vi "Condition ROI data.vi"(8 "error in (no error)":errorcluster, 9 "ROI numbers":i32[](array[numeric]), 10 "Data for ticked ROI":T1=[{"Plot.Plot Name"="1: Point", "Data"={"X-Axis values"=array[43860 elements], "Y-Axis values (s)"=array[43860 elements]}, "Timeline data"={"X-Axis values"=[], "Y-Axis values (s)"=[]}, "Type"=enum."Mini-scan", "Points per cycle"=1, "ROI number"=0}]) -> (0 "error out":errorcluster, 2 "Sorted Pointers":i32[](array[numeric]), 3 "Data reference":refnum<data-value>)   [LabVIEW 2013]
uses:
  xcontrol/Interface VIs/Interface typedefs/Interface-Data array.ctl
  xcontrol/Interface VIs/Interface typedefs/Interface-Data format definition.ctl
  xcontrol/Typedefs/Xctl-XY data type definition.ctl
  xcontrol/Typedefs/Xctrl-ROI type enum.ctl
  xcontrol/XGrapher.xctl
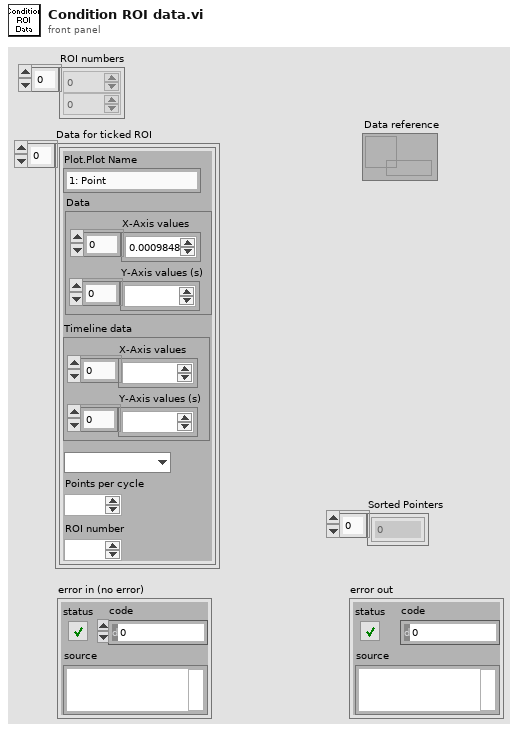
[diagram p1: front panel]
types:
  T1 = typedef "Interface-Data array.ctl" = T2[]
  T2 = typedef "Interface-Data format definition.ctl" = cluster{"Plot.Plot Name":string, "Data":T3, "Timeline data":T3, "Type":T4, "Points per cycle":u16, "ROI number":u16}
  T3 = typedef "XGrapher.xctl/Xctl-XY data type definition.ctl" = cluster{"X-Axis values":sgl[], "Y-Axis values (s)":i32[]}
  T4 = typedef "Xctrl-ROI type enum.ctl" = enum16{"POI", "Mini-scan", "Group"}
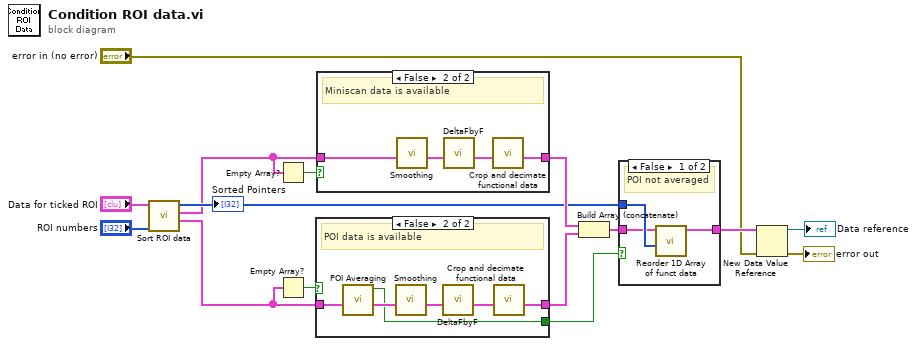
[diagram p0: block diagram]
diagram:
  n1 = call "Sort ROI data.vi"("ROI numbers"="ROI numbers", "Data for ticked ROI"="Data for ticked ROI") -> ("POI raw data"=w4:T1, "Miniscan raw data"=w3:T1, "Sorted Pointers"=w5:i32[])  [unwired: 7 in]
  "Sorted Pointers" <- w5
  n2 = Empty Array?(array=w3) -> (empty?=w11:bool)
  n3 = Empty Array?(array=w4) -> (empty?=w10:bool)
  n4 = case shown="False" w10 {
    tunnel: w4 -> [w16 w20]
    tunnel: [w16 w17] -> w13
    tunnel: [_ w19] -> w15
    frame True {
      # "No POI data available"
    }
    frame False {
      # "POI data is available"
      n5 = call "POI Averaging.vi"("Data in"=w20) -> ("Data out"=w21:T1, "Averaged"=w19:bool)  [unwired: 9 in]
      n6 = call "Smoothing.vi"("Data in"=w21) -> ("Data out"=w22:T1)  [unwired: 10 in]
      n7 = call "DeltaFbyF.vi"("Data in"=w22) -> ("Data out"=w18:T1)  [unwired: 10 in]
      n8 = call "Crop and decimate functional data.vi"("Data in"=w18) -> ("Data out"=w17:T1)  [unwired: 10 in]
    }
  }
  n9 = case shown="False" w11 {
    tunnel: w3 -> [w23 w26]
    tunnel: [w23 w24] -> w12
    frame True {
      # "No miniscan data available"
    }
    frame False {
      # "Miniscan data is available"
      n10 = call "Smoothing.vi"("Data in"=w26) -> ("Data out"=w27:T1)  [unwired: 10 in]
      n11 = call "DeltaFbyF.vi"("Data in"=w27) -> ("Data out"=w25:T1)  [unwired: 10 in]
      n12 = call "Crop and decimate functional data.vi"("Data in"=w25) -> ("Data out"=w24:T1)  [unwired: 10 in]
    }
  }
  n13 = Build Array (concatenate)(w12, w13) -> (w14:T1)
  n14 = case shown="False" w15 {
    tunnel: w5 -> [w30 _]
    tunnel: [w28 w31] -> w9
    tunnel: w14 -> [w29 w31]
    frame False {
      # "POI not averaged"
      n15 = call "Reorder 1D Array of funct data.vi"("indices"=w30, "Data in"=w29) -> ("Data out"=w28:T1)  [unwired: 9 in]
    }
    frame True {
      # "POI are averaged"
    }
  }
  n16 = New Data Value Reference(data value=w9, error in="error in (no error)") -> (data value reference=→"Data reference":refnum<data-value>, error out=→"error out":errorcluster)
